vi "Firmware_Version_Test.vi"() -> ()   [LabVIEW 2017]
panel:
  out "Test Result":picture
  out "XY Graph":cluster{dbl, u32}[](graph)
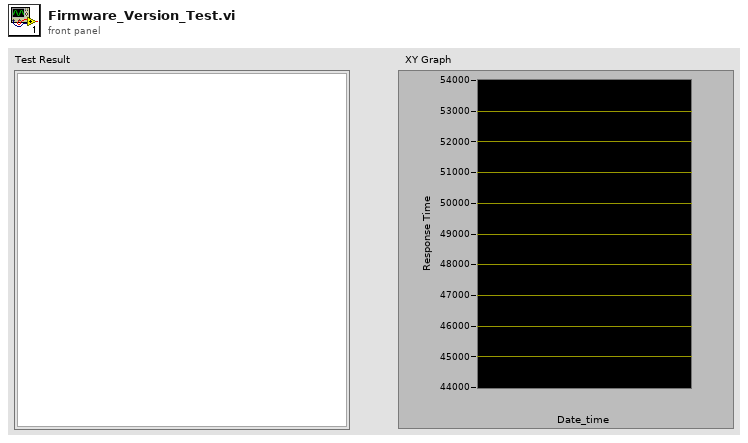
[diagram p1: front panel]
types:
  T1 = enum16{"open", "replace", "create", "open or create", "replace or create", "replace or create with confirmation"}
  T2 = cluster{"[0]":string, "[1]":string, "[2]":string, "[3]":string, "[4]":string, "[5]":string, "[6]":string, "[7]":string, "[8]":string}
  T3 = cluster{"Iterations":u64, "DelayBetweenIterations":u32, "Timeout":u32, "MessageID":i32, "MessageLength":i32, "ResponseID":i32, "Timestamp":string, "TestSuite":string, "ReportPath":path, "FWVersionPath":path}
  T4 = cluster{"Socket_IP_Address":string, "Socket_Port_Number":u16, "Global_ReportPath":path}
  T5 = typedef "imagedata.ctl" = cluster{"image type":i32, "image depth":i32, "image":u8[], "mask":u8[], "colors":u32[], "Rectangle":cluster{"left":i16, "top":i16, "right":i16, "bottom":i16}}
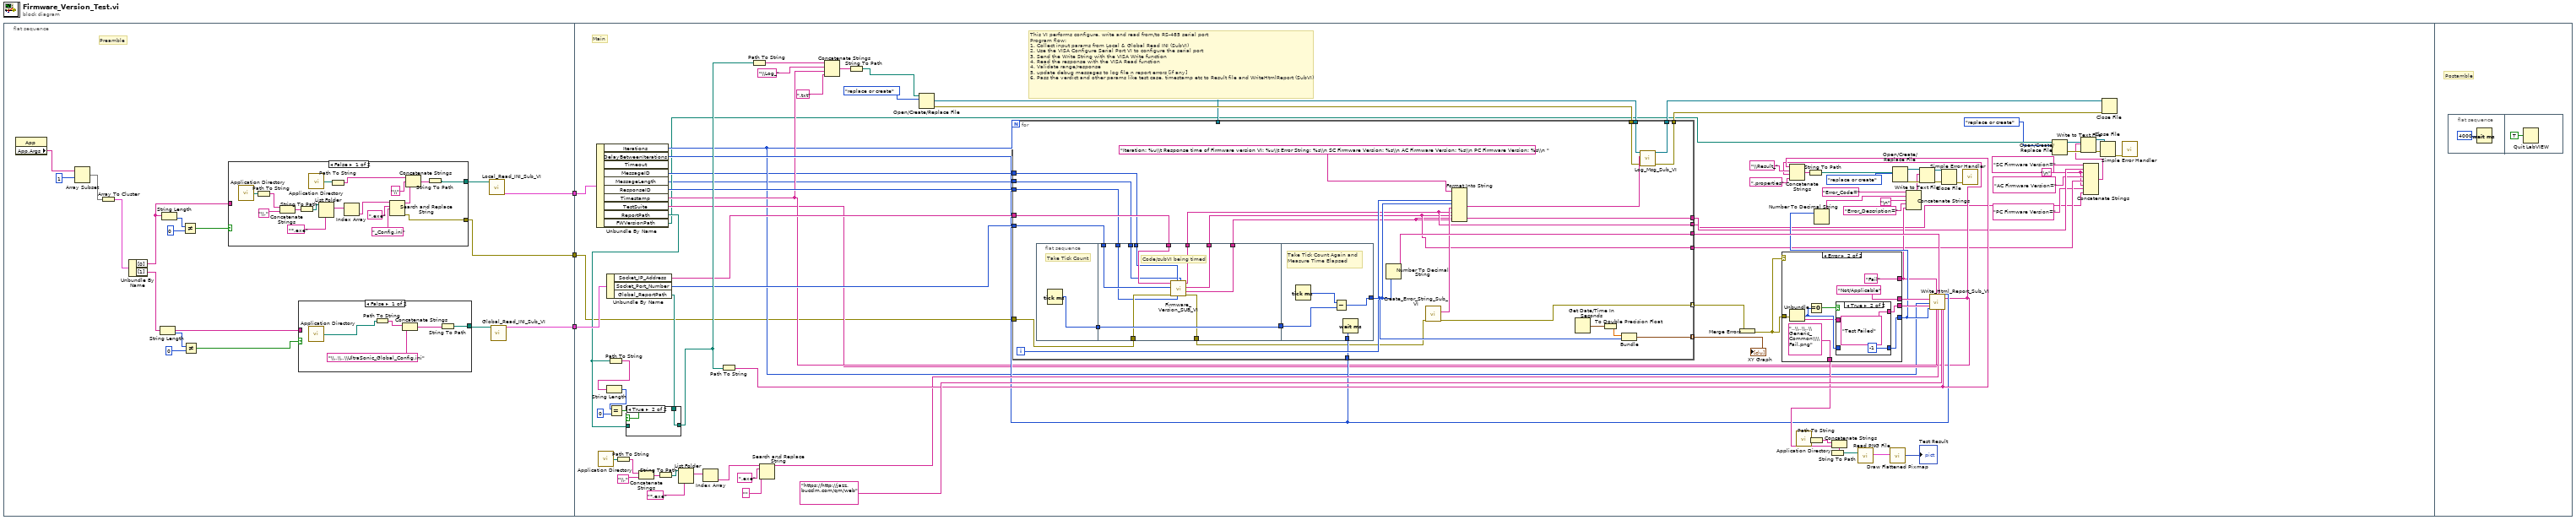
[diagram p0: block diagram]
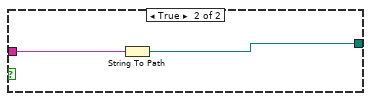
[diagram p2: hidden frame]
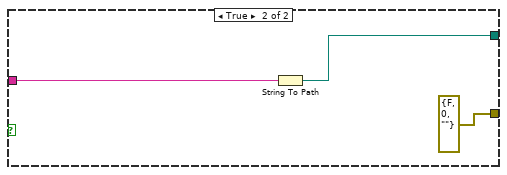
[diagram p3: hidden frame]
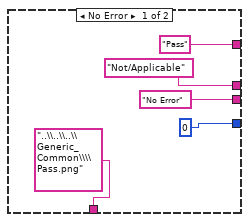
[diagram p5: hidden frame]
diagram:
  n1 = flat-sequence {
    tunnel: [w6] -> w3
    tunnel: [w5] -> w2
    tunnel: [w4] -> w1
    tunnel: w3 -> [w65]
    tunnel: w2 -> [w77]
    tunnel: w1 -> [w73]
    frame #0 {
      # "Preamble"
      n2 = property class="App"() -> ("App.Args"=w8:string[])  [unwired: 2 in, 2 out]
      n3 = Array Subset "Array Subset"(array=w8, index=1) -> (w9:string[])  [unwired: 1 in]
      n4 = Array To Cluster(array=w9) -> (cluster=w10:T2)
      n5 = Unbundle By Name "Unbundle By Name"(w10) -> ("[0]"=w14:string, "[1]"=w17:string)
      n6 = String Length(string=w17) -> (length=w18:i32)
      n7 = String Length(string=w14) -> (length=w11:i32)
      n8 = Not Equal?(x=w11, y=0) -> (x != y?=w13:bool)
      n9 = Not Equal?(x=w18, y=0) -> (x != y?=w16:bool)
      n10 = case shown="False" w13 {
        tunnel: w14 -> [_ w47]
        tunnel: [w29 w46] -> w19
        tunnel: [w28 errorcluster {"status"=FALSE, "code"=0, "source"=""} ("error out")] -> w6
        frame False {
          n11 = call <vilib>:"Application Directory.vi"() -> ("Application Directory"=w35:path)
          n12 = Path To String(path=w35) -> (string=w34:string)
          n13 = Concatenate Strings(w34, "\\." ("string")) -> (w32:string)
          n14 = String To Path(string=w32) -> (path=w37:path)
          n15 = call <vilib>:"Application Directory.vi"() -> ("Application Directory"=w44:path)
          n16 = List Folder(path=w37, pattern="*.exe") -> (filenames=w31:string[])  [unwired: 2 in, 3 out]
          n17 = Path To String(path=w44) -> (string=w39:string)
          n18 = Index Array(array=w31) -> (element=w30:string)  [unwired: 1 in]
          n19 = Search and Replace String(input string=w30, search string=".exe", replace string="_Config.ini" ("replace string (\"\")")) -> (result string=w41:string, error out=w28:errorcluster)  [unwired: 5 in, 2 out]
          n20 = Concatenate Strings(w39, "\\" ("string"), w41) -> (w38:string)
          n21 = String To Path(string=w38) -> (path=w29:path)
        }
        frame True {
          n22 = String To Path(string=w47) -> (path=w46:path)
        }
      }
      n23 = case shown="False" w16 {
        tunnel: [w22 w27] -> w20
        tunnel: w17 -> [_ w26]
        frame False {
          n24 = call <vilib>:"Application Directory.vi"() -> ("Application Directory"=w21:path)
          n25 = Path To String(path=w21) -> (string=w25:string)
          n26 = Concatenate Strings(w25, "\\..\\..\\UltraSonic_Global_Config.ini" ("string")) -> (w23:string)
          n27 = String To Path(string=w23) -> (path=w22:path)
        }
        frame True {
          n28 = String To Path(string=w26) -> (path=w27:path)
        }
      }
      n29 = call "Local_Read_INI_Sub_VI.vi"("Config File Path"=w19) -> ("output cluster"=w4:T3)  [unwired: 10 in]
      n30 = call "Global_Read_INI_Sub_VI.vi"("Config File Path"=w20) -> ("output cluster"=w5:T4)  [unwired: 14 in]
    }
    frame #1 {
      w51 = "\n"
      # "This VI performs configure, write and read from/to RS-485 serial port\nProgram flow:\n1. Collect input params from Local & Global Read INI (SubVI)\n2. Use the VISA Configure Serial Port VI to configure the serial port\n3. Send the Write String with the VISA Write function\n4. Read the response with the VISA Read function\n4. Validate range/response\n5. update debug messages to log file n report errors [if any]\n6. Pass the verdict and other params like test case, timestamp etc to Result file and WriteHtmlReport (SubVI)"
      # "Main"
      n31 = Unbundle By Name(w73) -> ("Iterations"=w67:u64, "DelayBetweenIterations"=w71:u32, "MessageID"=w64:i32, "MessageLength"=w48:i32, "ResponseID"=w72:i32, "Timestamp"=w69:string, "TestSuite"=w68:string, "ReportPath"=w66:path, "FWVersionPath"=w57:path)  [unwired: 1 out]
      n32 = call <vilib>:"Application Directory.vi"() -> ("Application Directory"=w93:path)
      n33 = Unbundle By Name(w77) -> ("Socket_IP_Address"=w75:string, "Socket_Port_Number"=w74:u16, "Global_ReportPath"=w76:path)
      n34 = Path To String(path=w66) -> (string=w124:string)
      n35 = String Length(string=w124) -> (length=w123:i32)
      n36 = Equal?(x=w123, y=0) -> (x = y?=w121:bool)
      n37 = Path To String(path=w93) -> (string=w92:string)
      n38 = case shown="True" w121 {
        tunnel: w76 -> [_ w136]
        tunnel: [w135 w136] -> w120
        tunnel: w66 -> [w135 _]
        frame False {
        }
        frame True {
        }
      }
      n39 = Concatenate Strings(w92, "\\." ("string")) -> (w90:string)
      n40 = String To Path(string=w90) -> (path=w95:path)
      n41 = List Folder(path=w95, pattern="*.exe") -> (filenames=w89:string[])  [unwired: 2 in, 3 out]
      n42 = Index Array(array=w89) -> (element=w85:string)  [unwired: 1 in]
      n43 = Path To String(path=w120) -> (string=w97:string)
      n44 = Path To String(path=w120) -> (string=w126:string)
      n45 = Search and Replace String(input string=w85, search string=".exe", replace string="" ("replace string (\"\")")) -> (result string=w88:string)  [unwired: 5 in, 3 out]
      n46 = Concatenate Strings(w126, "\\Log_" ("string"), w69, ".txt" ("string")) -> (w129:string)
      n47 = String To Path(string=w129) -> (path=w128:path)
      n48 = Open/Create/Replace File(file path (use dialog)=w128, operation (0:open)=T1."replace or create") -> (refnum out=w98:refnum<file>, error out=w101:errorcluster)  [unwired: 1 in, 4 out]
      n49 = for {
        N: w67 -> [_]
        tunnel: [w161] -> w132
        tunnel: w98 -> [w155]
        tunnel: [w154] -> w100
        tunnel: [w152] -> w99
        tunnel: [w157] -> w130 mode=indexing
        tunnel: w101 -> [w153]
        tunnel: w98 -> [_]
        tunnel: [w149] -> w96 mode=indexing
        tunnel: w75 -> [w148]
        tunnel: w74 -> [w147]
        tunnel: w72 -> [w145]
        tunnel: w71 -> [w146]
        tunnel: w65 -> [w144]
        tunnel: w64 -> [w143]
        tunnel: [w140] -> w54
        tunnel: [w139] -> w52
        tunnel: [w138] -> w49
        tunnel: w48 -> [w137]
        i -> [w150]
        n50 = flat-sequence {
          tunnel: [w164] -> w163
          tunnel: [w175] -> w162
          tunnel: w163 -> [w175]
          tunnel: w148 -> [w174]
          tunnel: w147 -> [w173]
          tunnel: w145 -> [w170]
          tunnel: w144 -> [w172]
          tunnel: w143 -> [w171]
          tunnel: [w169] -> w142
          tunnel: [w168] -> w140
          tunnel: [w167] -> w139
          tunnel: [w166] -> w138
          tunnel: w137 -> [w165]
          tunnel: w162 -> [w179]
          tunnel: [w177] -> w151
          tunnel: w146 -> [w176]
          frame #0 {
            # "Take Tick Count"
            n51 = Tick Count (ms)() -> (millisecond timer value=w164:u32)
          }
          frame #1 {
            # "Code/subVI being timed"
            n52 = call "Firmware_Version_SUB_VI.vi"("Message Length"=w165, "Firmware Response ID"=w170, "Firmware Request ID"=w171, "error in (no error)"=w172, "remote port or service name"=w173, "address"=w174) -> ("error out"=w169:errorcluster, "PC Firmware Version"=w166:string, "AC Firmware Version"=w167:string, "SC Firmware Version"=w168:string)  [unwired: 2 in]
          }
          frame #2 {
            # "Take Tick Count Again and Measure Time Elapsed"
            n53 = Tick Count (ms)() -> (millisecond timer value=w178:u32)
            n54 = Subtract(x=w178, y=w179) -> (x-y=w177:u32)
            n55 = Wait (ms)(milliseconds to wait=w176) -> ()  [unwired: 1 out]
          }
        }
        n56 = Number To Decimal String(number=w151) -> (decimal integer string=w161:string)  [unwired: 1 in]
        n57 = call "Create_Error_String_Sub_VI.vi"("error in"=w142) -> ("error out"=w149:errorcluster, "Error String"=w141:string)  [unwired: 9 in]
        n58 = Format Into String(format string="Iteration: %u\\t Response time of Firmware version VI: %u\\t Error String: %s\\n SC Firmware Version: %s\\n AC Firmware Version: %s\\n PC Firmware Version: %s\\n ", w150, w151, w141, w140, w139, w138) -> (resulting string=w156:string)  [unwired: 2 in, 1 out]
        n59 = Get Date/Time In Seconds() -> (seconds since 1Jan1904=w158:timestamp)
        n60 = To Double Precision Float(number=w158) -> (double precision float=w159:dbl)
        n61 = Bundle "Bundle"(w159, w151) -> (w157:cluster{dbl, u32})  [unwired: 1 in]
        n62 = call "Log_Msg_Sub_VI.vi"("error in (no error)"=w153, "String"=w156, "Byte Stream File in"=w155) -> ("error out"=w152:errorcluster, "Byte Stream File out"=w154:refnum<file>)  [unwired: 7 in]
      }
      "XY Graph" <- w130
      n63 = Merge Errors "Merge Errors"(w96) -> (w70:errorcluster)
      n64 = case shown="Error" w70 {
        tunnel: ["Pass" "Fail"] -> w102
        tunnel: w70 -> [_ w191]
        tunnel: [0 ("code") w187] -> w106
        tunnel: ["No Error" ("source") w188] -> w134
        tunnel: ["Not/Applicable" "Not/Applicable"] -> w133
        tunnel: ["..\\..\\..\\Generic_Common\\\\Pass.png" ("string") "..\\..\\..\\Generic_Common\\\\Fail.png" ("string")] -> w78
        frame No Error {
        }
        frame Error {
          n65 = Unbundle(w191) -> ("code"=w189:i32, "source"=w185:string)  [unwired: 1 out]
          n66 = Equal To 0?(x=w189) -> (x = 0?=w186:bool)
          n67 = case shown="True" w186 {
            tunnel: [w195 -1 ("code")] -> w187
            tunnel: [w194 "Test Failed" ("source")] -> w188
            tunnel: w189 -> [w195 _]
            tunnel: w185 -> [w194 _]
            frame False {
            }
            frame True {
            }
          }
        }
      }
      n68 = Concatenate Strings(w97, "\\Result_" ("string"), w69, ".properties" ("string")) -> (w118:string)
      n69 = call <vilib>:"Application Directory.vi"() -> ("Application Directory"=w79:path)
      n70 = String To Path(string=w118) -> (path=w110:path)
      n71 = Path To String(path=w79) -> (string=w80:string)
      n72 = Number To Decimal String(number=w106) -> (decimal integer string=w105:string)  [unwired: 1 in]
      n73 = Concatenate Strings(w80, w78) -> (w81:string)
      n74 = String To Path(string=w81) -> (path=w84:path)
      n75 = call <vilib>:"Read PNG File.vi"("path to PNG file"=w84) -> ("image data"=w82:T5)  [unwired: 8 in, 2 out]
      n76 = call <vilib>:"Draw Flattened Pixmap.vi"("image data"=w82) -> ("new picture"=→"Test Result":picture)  [unwired: 8 in]
      n77 = Open/Create/Replace File(file path (use dialog)=w110, operation (0:open)=T1."replace or create") -> (refnum out=w109:refnum<file>, error out=w114:errorcluster)  [unwired: 4 in, 1 out]
      n78 = Concatenate Strings("Error_Code=" ("string"), w105, "\n", "Error_Description=" ("string"), w102) -> (w108:string)
      n79 = Write to Text File(file (use dialog)=w109, text=w108, error in=w114) -> (refnum out=w113:refnum<file>, error out=w112:errorcluster)  [unwired: 1 in, 1 out]
      n80 = call "Write_Html_Report_Sub_VI.vi"("ReprtPath"=w97, "Remarks"=w133, "Iterations"=w67, "Error Description"=w134, "Timestamp"=w69, "TestCase"=w88, "Verdict"=w102, "TestSuite"=w68, "Time taken to execute  test in msec"=w132, "JazzDashboardLink"="https://http://jazz.bucclm.com/qm/web" ("TestSuite"), "Delay Between Iterations"=w71, "Error Code"=w106) -> ()  [unwired: 8 in]
      n81 = Close File(refnum=w113, error in=w112) -> (error out=w111:errorcluster)  [unwired: 1 out]
      n82 = call <vilib>:"Simple Error Handler.vi"("error in (no error)"=w111) -> ()  [unwired: 4 in, 5 out]
      n83 = Open/Create/Replace File(file path (use dialog)=w57, operation (0:open)=T1."replace or create") -> (refnum out=w59:refnum<file>, error out=w63:errorcluster)  [unwired: 4 in, 1 out]
      n84 = Concatenate Strings("SC Firmware Version=" ("string"), w54, w51, "AC Firmware Version=" ("string"), w52, w51, "PC Firmware Version=" ("string"), w49) -> (w58:string)
      n85 = Write to Text File(file (use dialog)=w59, text=w58, error in=w63) -> (refnum out=w62:refnum<file>, error out=w61:errorcluster)  [unwired: 1 in, 1 out]
      n86 = Close File(refnum=w62, error in=w61) -> (error out=w60:errorcluster)  [unwired: 1 out]
      n87 = Close File(refnum=w100, error in=w99) -> ()  [unwired: 2 out]
      n88 = call <vilib>:"Simple Error Handler.vi"("error in (no error)"=w60) -> ()  [unwired: 4 in, 5 out]
    }
    frame #2 {
      # "Postamble"
      n89 = flat-sequence {
        frame #0 {
          n90 = Wait (ms)(milliseconds to wait=u32 4000) -> ()  [unwired: 1 out]
        }
        frame #1 {
          n91 = Quit LabVIEW(quit? (T)=TRUE) -> ()
        }
      }
    }
  }
